vi "NSRwProgramie.vi"() -> ()   [LabVIEW 2024]
panel:
  out "Inkrementowanie":dbl
  in  "Sumowana":dbl
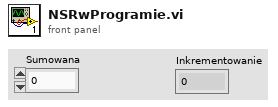
[diagram p1: front panel]
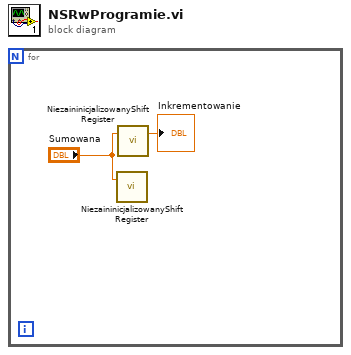
[diagram p0: block diagram]
diagram:
  n1 = for {
    n2 = call "NiezaininicjalizowanyShiftRegister.vi"("Sumowana"="Sumowana") -> ()  [unwired: 1 in, 2 out]
    n3 = call "NiezaininicjalizowanyShiftRegister.vi"("Sumowana"="Sumowana") -> ("Inkrementowanie"=→"Inkrementowanie":dbl)  [unwired: 1 in, 1 out]
  }
